vi "Local Variables.vi"() -> ()   [LabVIEW 2019]
doc: "This VI creates two queues to pass data between parallel loops. Queues are most useful when you need to send data from one or more data sources to one data sink with no potential loss of data."
panel:
  out "Received Data":dbl(graph)
  out "Generated Data":dbl(graph)
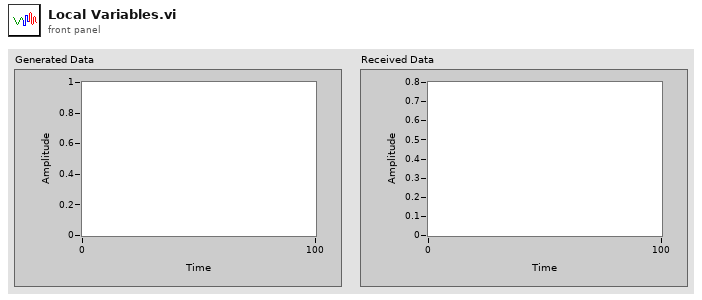
[diagram p1: front panel]
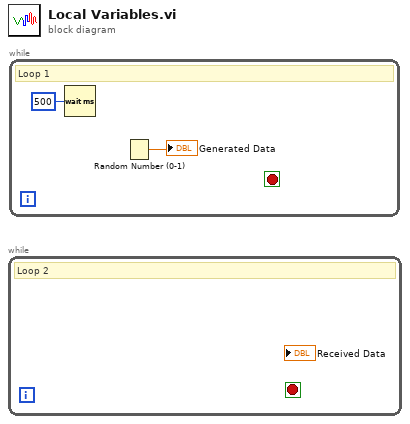
[diagram p0: block diagram]
diagram:
  n1 = while {
    stop <- _ stop-if-true
    # "Loop 2"
  }
  n2 = while {
    stop <- _ stop-if-true
    # "Loop 1"
    n3 = Wait (ms)(milliseconds to wait=u32 500) -> ()  [unwired: 1 out]
    n4 = Random Number (0-1)() -> (number: 0 to 1=→"Generated Data":dbl)
  }
